vi "Begin Cals.vi"() -> ()   [LabVIEW 2014]
panel:
  in  "Encoder Distance Per Rotation":dbl
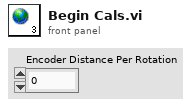
[diagram p1: front panel]
diagram:
